vi "SelectChip.vi"(8 "error in (no error)":errorcluster, 10 "chipSelection":string="LT9611", 11 "LT_UpgradeFlash in":refnum<class "LT_UpgradeFlash.lvclass">) -> (0 "error out":errorcluster, 1 "resultStr":string, 2 "ActionResult":bool, 3 "LT_UpgradeFlash out":refnum<class "LT_UpgradeFlash.lvclass">)   [LabVIEW 2017, in "LT_UpgradeFlash.lvclass"]
uses:
  LT_UpgradeFlash.lvclass
  D:/Project/Tymphany/LT_UpgradeFlash/New_Lib/LT_UpgradeFlash_dll/LT_UpgradeFlash_dll/bin/Debug/LT_UpgradeFlash_dll.dll
  New_Lib/LT_UpgradeFlash_dll/LT_UpgradeFlash_dll/bin/Debug/LT_UpgradeFlash_dll.dll
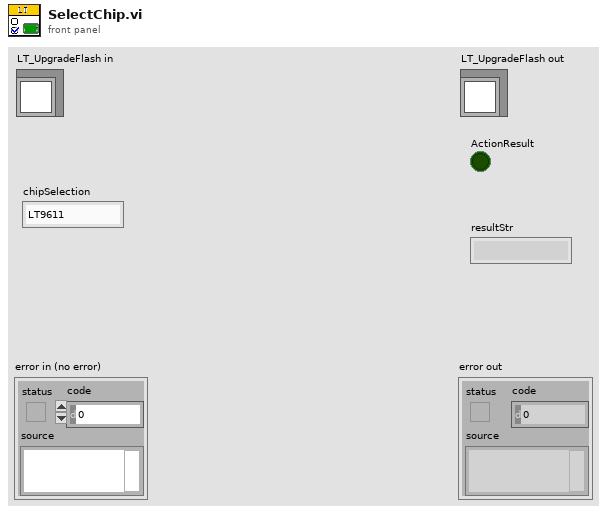
[diagram p1: front panel]
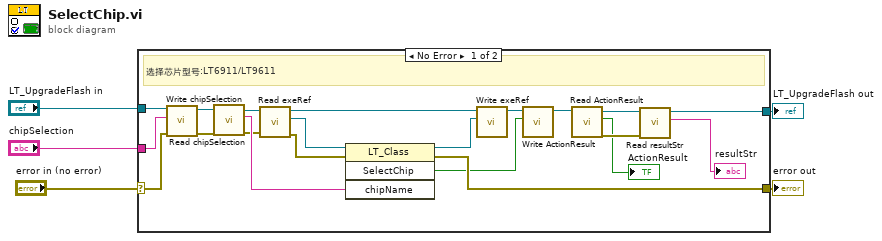
[diagram p0: block diagram]
diagram:
  n1 = case shown="No Error" "error in (no error)" {
    selector: "error in (no error)" -> [w12 w28]
    tunnel: [w23 w28] -> w4
    tunnel: [w7 w27] -> w2
    tunnel: "LT_UpgradeFlash in" -> [w16 w27]
    tunnel: "chipSelection" -> [w13 _]
    frame No Error {
      # "选择芯片型号:LT6911/LT9611"
      n2 = call-dynamic "Write chipSelection.vi"("error in (no error)"=w12, "chipSelection"=w13, "LT_UpgradeFlash in"=w16) -> ("error out"=w14:errorcluster, "LT_UpgradeFlash out"=w15:refnum<class "LT_UpgradeFlash.lvclass">)  [unwired: 7 in]
      n3 = call-dynamic "Read chipSelection.vi"("error in (no error)"=w14, "LT_UpgradeFlash in"=w15) -> ("error out"=w18:errorcluster, "chipSelection"=w25:string, "LT_UpgradeFlash out"=w24:refnum<class "LT_UpgradeFlash.lvclass">)  [unwired: 7 in]
      n4 = call-dynamic "Read exeRef.vi"("error in (no error)"=w18, "LT_UpgradeFlash in"=w24) -> ("error out"=w17:errorcluster, "exeRef"=w26:refnum<k24>, "LT_UpgradeFlash out"=w22:refnum<class "LT_UpgradeFlash.lvclass">)  [unwired: 7 in]
      n5 = invoke class="LT_Class" method="SelectChip"(reference=w26, error in=w17, "chipName"=w25) -> (reference out=w20:refnum<k24>, error out=w23:errorcluster, "SelectChip"=w19:bool)  [unwired: 1 in, 1 out]
      n6 = call-dynamic "Write exeRef.vi"("exeRef"=w20, "LT_UpgradeFlash in"=w22) -> ("LT_UpgradeFlash out"=w21:refnum<class "LT_UpgradeFlash.lvclass">)  [unwired: 8 in, 1 out]
      n7 = call-dynamic "Write ActionResult.vi"("ActionResult"=w19, "LT_UpgradeFlash in"=w21) -> ("LT_UpgradeFlash out"=w6:refnum<class "LT_UpgradeFlash.lvclass">)  [unwired: 8 in, 1 out]
      n8 = call-dynamic "Read ActionResult.vi"("LT_UpgradeFlash in"=w6) -> ("error out"=w10:errorcluster, "ActionResult"=→"ActionResult":bool, "LT_UpgradeFlash out"=w11:refnum<class "LT_UpgradeFlash.lvclass">)  [unwired: 8 in]
      n9 = call-dynamic "Read resultStr.vi"("error in (no error)"=w10, "LT_UpgradeFlash in"=w11) -> ("resultStr"=→"resultStr":string, "LT_UpgradeFlash out"=w7:refnum<class "LT_UpgradeFlash.lvclass">)  [unwired: 7 in, 1 out]
    }
    frame Error {
    }
  }
  "error out" <- w4
  "LT_UpgradeFlash out" <- w2
